vi "Cycling.vi"() -> ()   [LabVIEW 2020]
panel:
  in  "Number of Cycles":i32
  in  "Charge filepath":path
  in  "Discharge filepath":path
  in  "Batteryname":string
  in  "Starting Cycle":i32
  out "PS error out":errorcluster
  out "PS Visa Out":refnum<visa-resource-name>
  out "parallel task error out":errorcluster
  out "parallel task out":refnum<k21>
  in  "Wait time":dbl
  in  "Discharge Current Setpoint":dbl format="%#.6g"
  in  "Charge Current Setpoint":dbl format="%#.6g"
  in  "Battery Type":enum16{"30Q", "40T"}(ring)
  in  "PS type":enum16{"NHR", "ITECH"}(ring)
  in  "#DAQ outputs (1-13)":i32
  in  "Data Task in":refnum<k21>
  in  "data task error in":errorcluster
  in  "PS error in":errorcluster caption="PS error in (no error)"
  in  "PS VISA in":refnum<visa-resource-name>
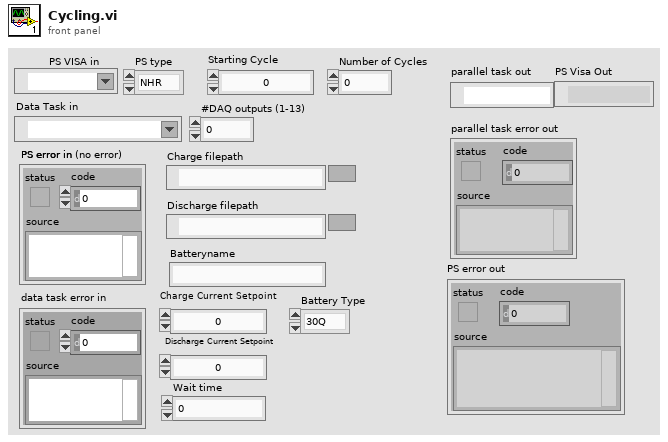
[diagram p1: front panel]
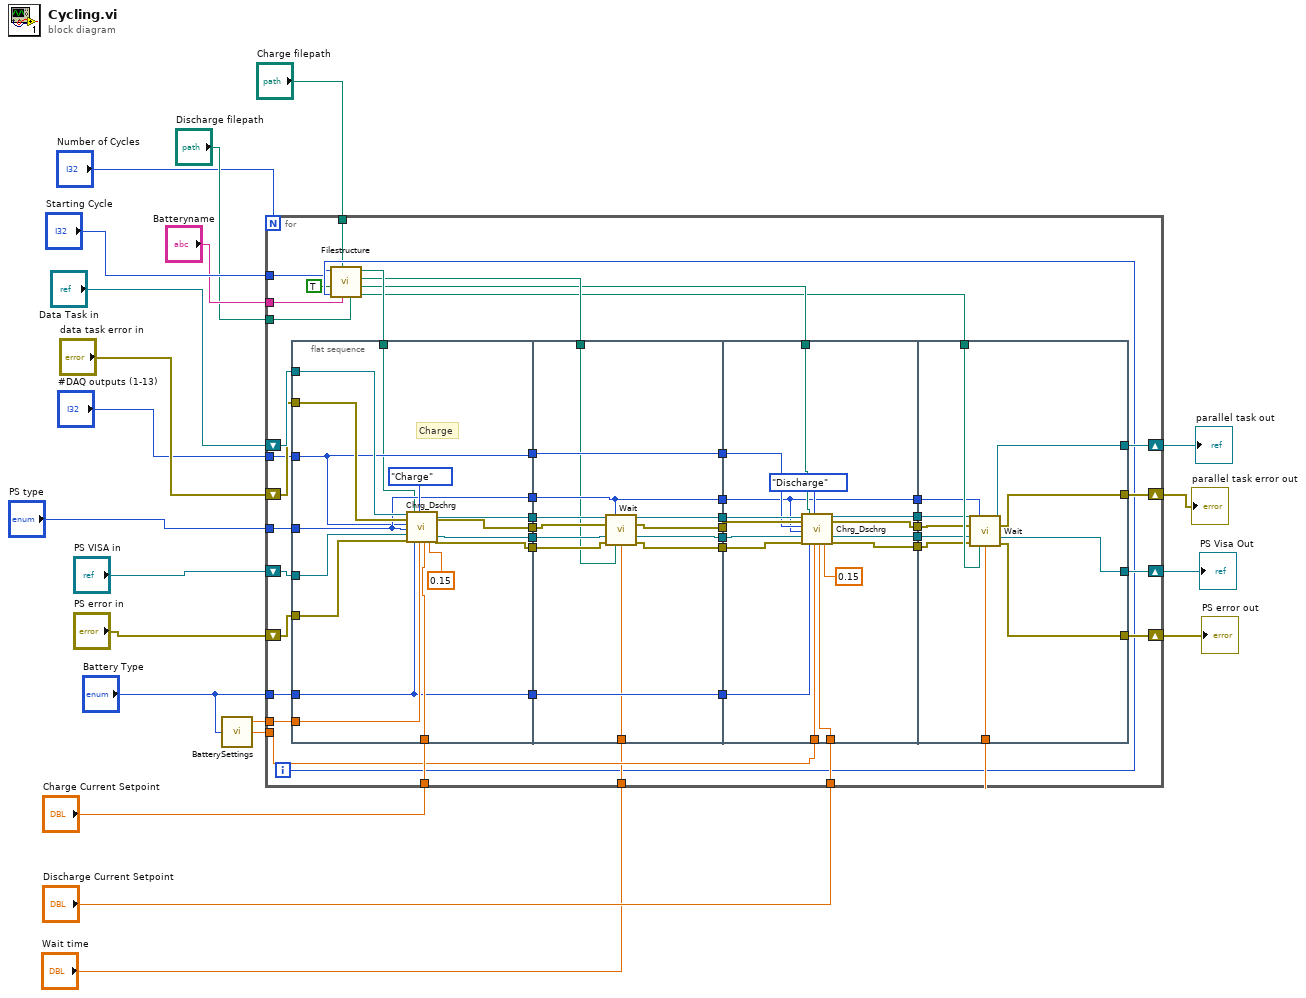
[diagram p0: block diagram]
diagram:
  n1 = call "BatterySettings.vi"("Battery Type"="Battery Type") -> ("Min Voltage (V)"=w12:dbl, "Max Voltage (V)"=w15:dbl)  [unwired: 2 in, 1 out]
  n2 = for {
    N: "Number of Cycles" -> [_]
    tunnel: "#DAQ outputs (1-13)" -> [w45]
    tunnel: "PS type" -> [w44]
    tunnel: w15 -> [w41]
    tunnel: "Battery Type" -> [w40]
    tunnel: "Charge Current Setpoint" -> [w39]
    tunnel: w12 -> [w38]
    tunnel: "Discharge Current Setpoint" -> [w37]
    tunnel: "Wait time" -> [w32]
    shift-right: [w28] -> w6
    shift-left: "Data Task in" -> [w47]
    shift-right: [w29] -> w7
    shift-left: "data task error in" -> [w46]
    shift-right: [w30] -> w8
    shift-left: "PS VISA in" -> [w43]
    shift-right: [w31] -> w9
    shift-left: "PS error in" -> [w42]
    tunnel: "Starting Cycle" -> [w26]
    tunnel: "Batteryname" -> [w24]
    tunnel: "Discharge filepath" -> [w23]
    tunnel: "Charge filepath" -> [w22]
    i -> [w27]
    n3 = flat-sequence {
      tunnel: w47 -> [w82]
      tunnel: w46 -> [w81]
      tunnel: w45 -> [w69]
      tunnel: w44 -> [w70]
      tunnel: w43 -> [w80]
      tunnel: w42 -> [w79]
      tunnel: w40 -> [w68]
      tunnel: w41 -> [w76]
      tunnel: w39 -> [w75]
      tunnel: [w74] -> w66
      tunnel: [w73] -> w65
      tunnel: [w72] -> w64
      tunnel: [w71] -> w63
      tunnel: [w70] -> w62
      tunnel: [w69] -> w61
      tunnel: [w68] -> w60
      tunnel: w36 -> [w67]
      tunnel: w66 -> [w95]
      tunnel: w65 -> [w94]
      tunnel: w64 -> [w93]
      tunnel: w63 -> [w92]
      tunnel: w62 -> [w86]
      tunnel: [w91] -> w59
      tunnel: [w90] -> w58
      tunnel: [w89] -> w57
      tunnel: [w88] -> w56
      tunnel: w61 -> [w87]
      tunnel: [w87] -> w55
      tunnel: [w86] -> w54
      tunnel: w60 -> [w85]
      tunnel: [w85] -> w53
      tunnel: w35 -> [w84]
      tunnel: w32 -> [w83]
      tunnel: w59 -> [w111]
      tunnel: w58 -> [w110]
      tunnel: w57 -> [w109]
      tunnel: w56 -> [w108]
      tunnel: w55 -> [w107]
      tunnel: w54 -> [w96]
      tunnel: w53 -> [w106]
      tunnel: w38 -> [w105]
      tunnel: w37 -> [w104]
      tunnel: w34 -> [w101]
      tunnel: [w100] -> w52
      tunnel: [w99] -> w51
      tunnel: [w98] -> w50
      tunnel: [w97] -> w49
      tunnel: [w96] -> w48
      tunnel: w33 -> [w122]
      tunnel: w52 -> [w121]
      tunnel: w51 -> [w120]
      tunnel: w50 -> [w119]
      tunnel: w49 -> [w118]
      tunnel: w32 -> [w117]
      tunnel: w48 -> [w116]
      tunnel: [w115] -> w31
      tunnel: [w114] -> w30
      tunnel: [w113] -> w29
      tunnel: [w112] -> w28
      frame #0 {
        # "Charge"
        n4 = call "Chrg_Dschrg.vi"("Data Task in"=w82, "data task error in"=w81, "#DAQ outputs (1-13)"=w69, "PS type"=w70, "PS VISA in"=w80, "PS error in"=w79, "CyclePath"=w67, "Battery Type"=w68, "Charge/discharge"=enum8{"Charge", "Discharge"}."Charge", "Charge/Discharge Voltage Setpoint"=w76, "Current Setpoint"=w75, "Current Cutoff"=0.15) -> ("data task out"=w74:refnum<k21>, "data task error out"=w73:errorcluster, "VISA resource name out"=w72:refnum<visa-resource-name>, "NHR error out"=w71:errorcluster)  [unwired: 4 in]
      }
      frame #1 {
        n5 = call "Wait.vi"("data Task in"=w95, "PS type"=w86, "data task error in"=w94, "PS VISA in"=w93, "PS error in"=w92, "Wait Filepath"=w84, "Wait time"=w83) -> ("parallel task out"=w91:refnum<k21>, "parallel task error out"=w90:errorcluster, "PS Visa Out"=w89:refnum<visa-resource-name>, "PS error out"=w88:errorcluster)  [unwired: 5 in]
      }
      frame #2 {
        n6 = call "Chrg_Dschrg.vi"("Data Task in"=w111, "data task error in"=w110, "#DAQ outputs (1-13)"=w107, "PS type"=w96, "PS VISA in"=w109, "PS error in"=w108, "CyclePath"=w101, "Battery Type"=w106, "Charge/discharge"=enum8{"Charge", "Discharge"}."Discharge", "Charge/Discharge Voltage Setpoint"=w105, "Current Setpoint"=w104, "Current Cutoff"=0.15) -> ("data task out"=w100:refnum<k21>, "data task error out"=w99:errorcluster, "VISA resource name out"=w98:refnum<visa-resource-name>, "NHR error out"=w97:errorcluster)  [unwired: 4 in]
      }
      frame #3 {
        n7 = call "Wait.vi"("data Task in"=w121, "PS type"=w116, "data task error in"=w120, "PS VISA in"=w119, "PS error in"=w118, "Wait Filepath"=w122, "Wait time"=w117) -> ("parallel task out"=w112:refnum<k21>, "parallel task error out"=w113:errorcluster, "PS Visa Out"=w114:refnum<visa-resource-name>, "PS error out"=w115:errorcluster)  [unwired: 5 in]
      }
    }
    n8 = call "Filestructure.vi"("Discharge filepath"=w23, "Batteryname"=w24, "Charge filepath"=w22, "For loop i"=w27, "In for loop"=TRUE, "Starting Cycle"=w26) -> ("DischargeWaitPath"=w33:path, "DischargeCyclePath"=w34:path, "ChargeWaitPath"=w35:path, "ChargeCyclePath"=w36:path)  [unwired: 1 in, 1 out]
  }
  "PS error out" <- w9
  "PS Visa Out" <- w8
  "parallel task error out" <- w7
  "parallel task out" <- w6
